vi "Capture GPS Waypoints.vi"() -> (0 "GPS Coordinates":cluster{"Latitude":dbl, "Longitude":dbl}[](array[cluster]))   [LabVIEW 2011]
uses:
  _GlobalVariables&Libraries/ATV Program Global Variables.vi
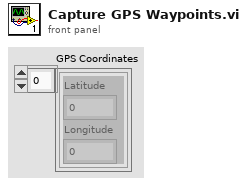
[diagram p1: front panel]
types:
  T1 = cluster{"Drive Value Output String":string, "Steer Value Output String":string, "Button A":bool, "Button B":bool, "Error Out":errorcluster, "Disable XBox Drive & Steer":bool, "Disable XBox Controller":bool, "XBOX Button Trigger Time (ms)":u32, "Button X":bool, "Button Y":bool}
  T2 = cluster{"GPS VISA resource name":refnum<visa-resource-name>, "GPS Error":errorcluster, "Disable GPS VISA":bool, "Latitude":dbl, "Longitude":dbl, "Latitude Uncertainty":dbl, "Longitude Uncertainty":dbl, "GPS Signal":u32}
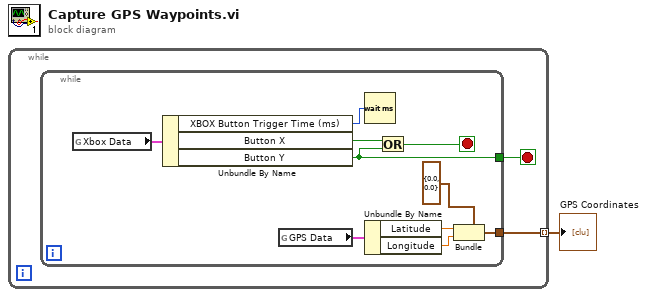
[diagram p0: block diagram]
diagram:
  n1 = while {
    tunnel: [w2] -> w1 mode=indexing
    stop <- w3 stop-if-true
    n2 = while {
      tunnel: [w4] -> w3
      tunnel: [w7] -> w2
      stop <- w6 stop-if-true
      n3 = global read "ATV Program Global Variables.vi" "Xbox Data"() -> (w13:T1)
      n4 = Unbundle By Name(w13) -> ("XBOX Button Trigger Time (ms)"=w12:u32, "Button X"=w5:bool, "Button Y"=w4:bool)
      n5 = global read "ATV Program Global Variables.vi" "GPS Data"() -> (w8:T2)
      n6 = Wait (ms)(milliseconds to wait=w12) -> ()  [unwired: 1 out]
      n7 = Unbundle By Name(w8) -> ("Latitude"=w10:dbl, "Longitude"=w11:dbl)
      n8 = Or(x=w5, y=w4) -> (x .or. y?=w6:bool)
      n9 = Bundle(cluster=cluster{"Latitude":dbl, "Longitude":dbl} {"Latitude"=0.0, "Longitude"=0.0} ("Cluster"), "Latitude"=w10, "Longitude"=w11) -> (w7:cluster{"Latitude":dbl, "Longitude":dbl})
    }
  }
  "GPS Coordinates" <- w1
